vi "regSubEvents.vi"(8 "error in (no error)":errorcluster, 11 "SALCommunicatorController in":refnum<class "SALCommunicatorController.lvclass">) -> (0 "error out":errorcluster, 2 "Event Registration Refnum":refnum<event-registration>, 3 "SALCommunicatorController out":refnum<class "SALCommunicatorController.lvclass">)   [LabVIEW 2016, in "SALCommunicatorController.lvclass"]
uses:
  SALCommunicatorController.lvclass
  <vilib>/Utility/error.llb/DialogType.ctl
  ts_sallv_exa/SALLV_EXA.lvlib
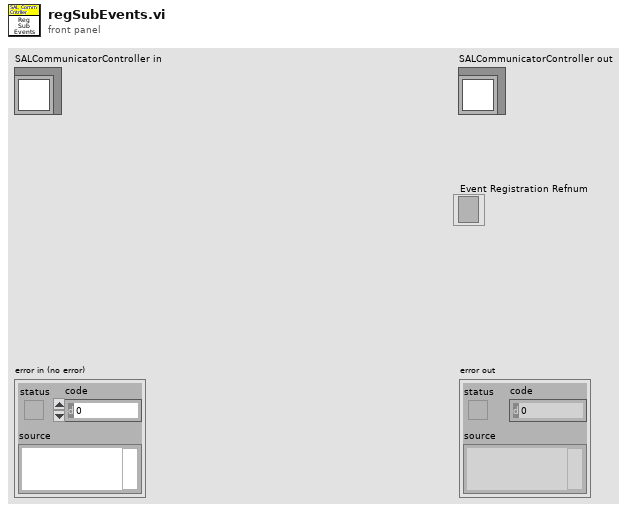
[diagram p1: front panel]
types:
  T1 = typedef "DialogType.ctl" = u16
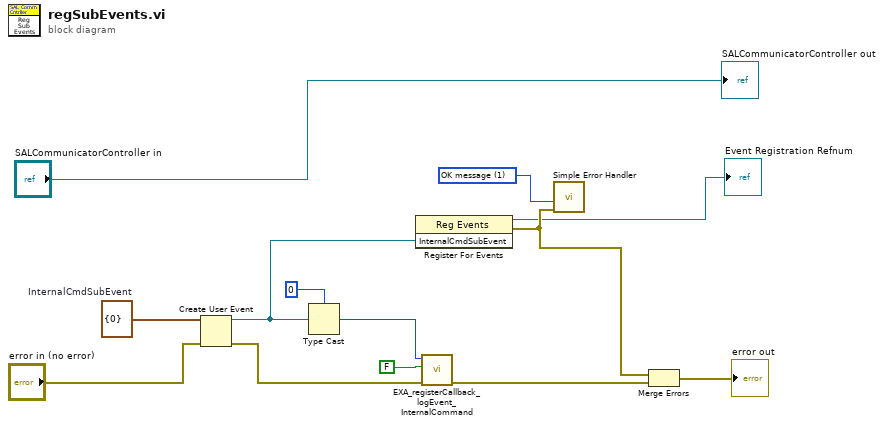
[diagram p0: block diagram]
diagram:
  w5 = cluster{"Data":i32} {"Data"=0}  # InternalCmdSubEvent
  w13 = T1 1 items=["no dialog", "OK message", "continue or stop message", "OK message + warnings", "continue/stop + warnings"] ("type of dialog (OK msg:1)")
  n1 = Create User Event(user event datatype=w5, error in="error in (no error)") -> (user event=w4:refnum<user-event>, error out=w1:errorcluster)
  n2 = Type Cast(type=0, x=w4) -> (*(type *) &x=w10:i32)
  n3 = register-events(w4) -> (reference out=→"Event Registration Refnum":refnum<event-registration>, error out=w7:errorcluster)  [unwired: 2 in]
  n4 = call "EXA_registerCallback_logEvent_InternalCommand.vi"("error in (no error)"=w1, "skipOld"=FALSE, "handle"=w10) -> ("error out"=w6:errorcluster)  [unwired: 7 in, 1 out]
  n5 = call <vilib>:"Simple Error Handler.vi"("type of dialog (OK msg:1)"=w13, "error in (no error)"=w7) -> ()  [unwired: 3 in, 5 out]
  n6 = Merge Errors(w7, w6) -> (→"error out":errorcluster)
  "SALCommunicatorController out" <- "SALCommunicatorController in"
